vi "DXD Pressure Sensors Control.vi"(9 "Record Pressure?":bool, 11 "Slave Data Cluster":T1={"Current DoE"=[], "SSI 1 Flow Rate"=0.0, "SSI 2 Flow Rate"=0.0, "FLOM 1 Flow Rate"=0.0, "FLOM 2 Flow Rate"=0.0, "Pumps Running?"=FALSE, "Boolean 2"=FALSE, "Boolean 3"=FALSE, "Boolean 4"=FALSE, "At Equilibrium?"=FALSE, "Script Running?"=FALSE, "Current Script Iteration"=0.0, "Total Script Iterations"=0.0, "FLOM Pumps VISA"="COM2", "SSI 1 Pump VISA"="COM76", "SSI 2 Pump VISA"="COM74", "Huber Unistat VISA"="COM1", "SSI 3 Pump VISA"="COM76", "SSI 4 Pump VISA"="COM76", "SSI 4 Flow Rate"=0.0, "SSI 3 Flow Rate"=0.0, "Flow Meter 1 Rate "=0.0, "Flow Meter 2 Rate"=0.0, "Flow Meter 3 Rate"=0.0, "Flow Meter 4 Rate"=0.0, "SSI 1 Flow Setpoint"=0.0, "SSI 2 Flow Setpoint"=0.0, "SSI 3 Flow Setpoint"=0.0, "SSI 4 Flow Setpoint"=0.0, "Temperature Setpoint"=0.0, "Flow meter 3 COM"=17, "Flow meter 5 COM"=18, "Flow meter 4 COM"=19, "Flow meter 2 COM"=16, "Flow meter 1 COM"=15, "Unit"=enum."PSI", "Pressure COM"="COM6"} {"Current DoE" format="%0.3f"}) -> (1 "Temperature Plot":T3, 2 "PressurePlot":T2, 3 "Pressure Data Out to Write":T2)   [LabVIEW 2015]
uses:
  --Controls and TypeDefs--/DoE_Control_Cluster.ctl
  --Sensor and Instrument Drivers--/LabView VI Drivers for Heise DXD Digital Pressure Transducer/Type Defs/DXD Address.ctl
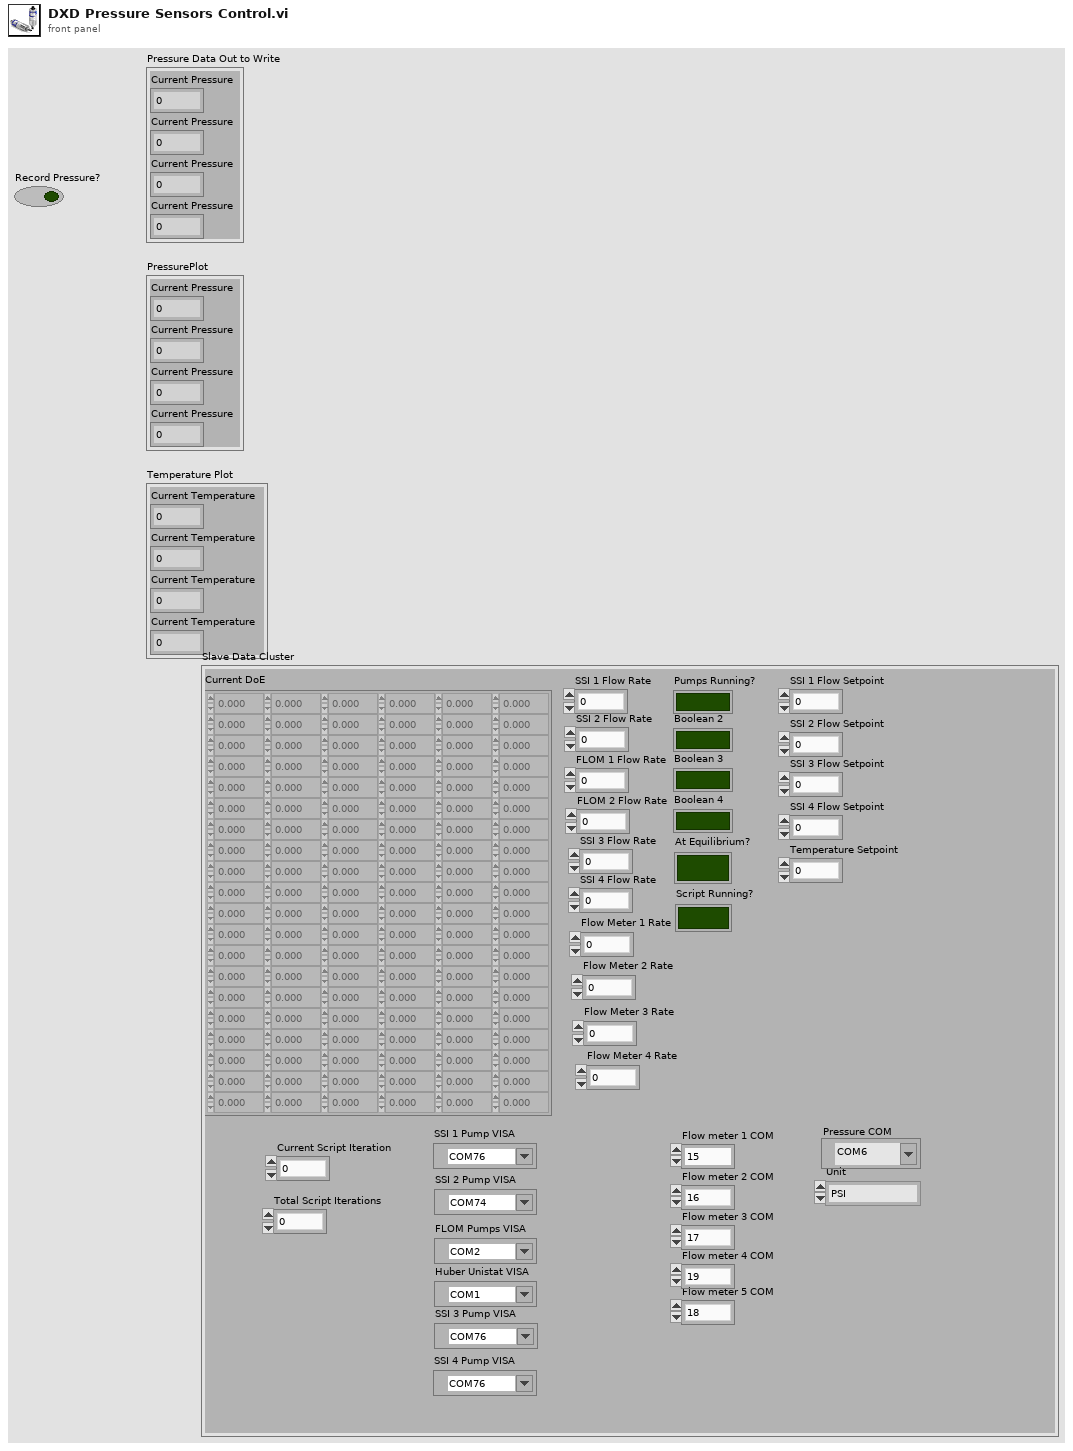
[diagram p1: front panel]
types:
  T1 = typedef "DoE_Control_Cluster.ctl" = cluster{"Current DoE":dbl[][], "SSI 1 Flow Rate":dbl, "SSI 2 Flow Rate":dbl, "FLOM 1 Flow Rate":dbl, "FLOM 2 Flow Rate":dbl, "Pumps Running?":bool, "Boolean 2":bool, "Boolean 3":bool, "Boolean 4":bool, "At Equilibrium?":bool, "Script Running?":bool, "Current Script Iteration":dbl, "Total Script Iterations":dbl, "FLOM Pumps VISA":refnum<visa-resource-name>, "SSI 1 Pump VISA":refnum<visa-resource-name>, "SSI 2 Pump VISA":refnum<visa-resource-name>, "Huber Unistat VISA":refnum<visa-resource-name>, "SSI 3 Pump VISA":refnum<visa-resource-name>, "SSI 4 Pump VISA":refnum<visa-resource-name>, "SSI 4 Flow Rate":dbl, "SSI 3 Flow Rate":dbl, "Flow Meter 1 Rate ":dbl, "Flow Meter 2 Rate":dbl, "Flow Meter 3 Rate":dbl, "Flow Meter 4 Rate":dbl, "SSI 1 Flow Setpoint":dbl, "SSI 2 Flow Setpoint":dbl, "SSI 3 Flow Setpoint":dbl, "SSI 4 Flow Setpoint":dbl, "Temperature Setpoint":dbl, "Flow meter 3 COM":u16, "Flow meter 5 COM":u16, "Flow meter 4 COM":u16, "Flow meter 2 COM":u16, "Flow meter 1 COM":u16, "Unit":enum16{"PSI", "Bar", "cm H2O", "ft H2O", "hectoPascal", "in Hg", "in H2O", "kiloPascal", "milliBar", "mmHg", "MegaPascal", "Numeric Pressure"}, "Pressure COM":refnum<visa-resource-name>}
  T2 = cluster{"Current Pressure":dbl, "Current Pressure":dbl, "Current Pressure":dbl, "Current Pressure":dbl}
  T3 = cluster{"Current Temperature":dbl, "Current Temperature":dbl, "Current Temperature":dbl, "Current Temperature":dbl}
  T4 = enum16{"PSI", "Bar", "cm H2O", "ft H2O", "hectoPascal", "in Hg", "in H2O", "kiloPascal", "milliBar", "mmHg", "MegaPascal", "Numeric Pressure"}
  T5 = typedef "DXD Address.ctl" = i32
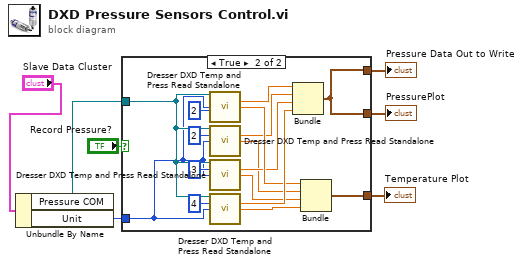
[diagram p0: block diagram]
diagram:
  n1 = Unbundle By Name("Slave Data Cluster") -> ("Pressure COM"=w1:refnum<visa-resource-name>, "Unit"=w2:T4)
  n2 = case shown="True" "Record Pressure?" {
    tunnel: [_ w10] -> w4
    tunnel: [_ w11] -> w6
    tunnel: [_ w10] -> w7
    tunnel: w1 -> [_ w9]
    tunnel: w2 -> [_ w8]
    frame False {
    }
    frame True {
      n3 = call "Dresser DXD Temp and Press Read Standalone.vi"("Serial Port (COM1)"=w9, "DXD Address (1)"=T5 2, "Pressure Units (PSI)"=w8) -> ("Current Pressure"=w15:dbl, "Current Temperature"=w18:dbl)  [unwired: 9 in, 2 out]
      n4 = call "Dresser DXD Temp and Press Read Standalone.vi"("Serial Port (COM1)"=w9, "DXD Address (1)"=T5 2, "Pressure Units (PSI)"=w8) -> ("Current Pressure"=w16:dbl, "Current Temperature"=w14:dbl)  [unwired: 9 in, 2 out]
      n5 = call "Dresser DXD Temp and Press Read Standalone.vi"("Serial Port (COM1)"=w9, "DXD Address (1)"=T5 3, "Pressure Units (PSI)"=w8) -> ("Current Pressure"=w17:dbl, "Current Temperature"=w13:dbl)  [unwired: 9 in, 2 out]
      n6 = call "Dresser DXD Temp and Press Read Standalone.vi"("Serial Port (COM1)"=w9, "DXD Address (1)"=T5 4, "Pressure Units (PSI)"=w8) -> ("Current Pressure"=w19:dbl, "Current Temperature"=w12:dbl)  [unwired: 9 in, 2 out]
      n7 = Bundle("Current Pressure"=w15, "Current Pressure"=w16, "Current Pressure"=w17, "Current Pressure"=w19) -> (w10:T2)  [unwired: 1 in]
      n8 = Bundle("Current Temperature"=w18, "Current Temperature"=w14, "Current Temperature"=w13, "Current Temperature"=w12) -> (w11:T3)  [unwired: 1 in]
    }
  }
  "PressurePlot" <- w7
  "Temperature Plot" <- w6
  "Pressure Data Out to Write" <- w4
